vi "Start and End to Array.vi"(4 "Round Factor":dbl=1000000000.0, 5 "Step":dbl=0.1, 6 "End":dbl=2.0, 7 "Start":dbl=-0.5) -> (1 "Array":dbl[](array[numeric])=[-0.5, -0.4, -0.3, -0.2, -0.1, 0.0, 0.1, 0.2, 0.3, 0.4, 0.5, 0.6, 0.7, 0.8, 0.9, 1.0, 1.1, 1.2, 1.3, 1.4, 1.5, 1.6, 1.7, 1.8, 1.9, 2.0])   [LabVIEW 2010]
panel:
  in  "Sweep Style":enum16{"Linear", "Log"}(ring)
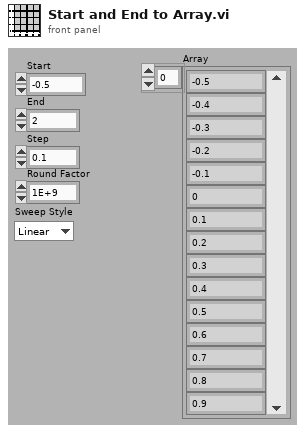
[diagram p1: front panel]
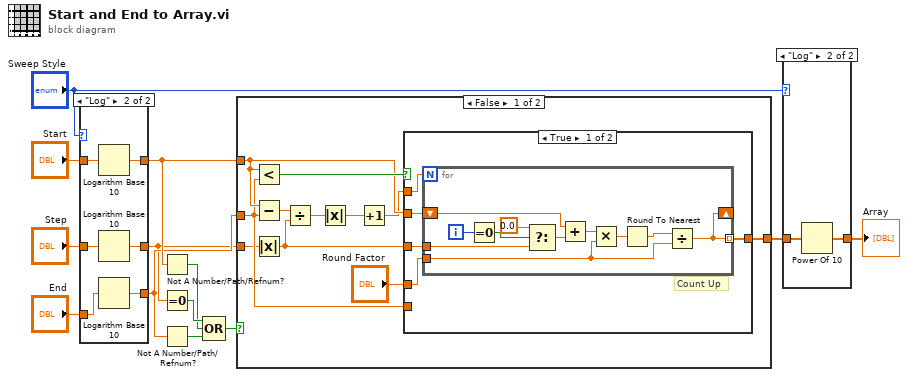
[diagram p0: block diagram]
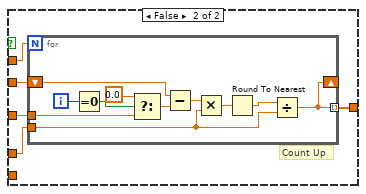
[diagram p4: hidden frame]
diagram:
  n1 = case shown="\"Log\"" "Sweep Style" {
    tunnel: "Start" -> [w16 w22]
    tunnel: [w16 w21] -> w8
    tunnel: "End" -> [w15 w18]
    tunnel: [w15 w17] -> w6
    tunnel: "Step" -> [w14 w20]
    tunnel: [w14 w19] -> w4
    frame "Linear", Default {
    }
    frame "Log" {
      n2 = Logarithm Base 10(1:w22) -> (0:w21:dbl)
      n3 = Logarithm Base 10(1:w20) -> (0:w19:dbl)
      n4 = Logarithm Base 10(1:w18) -> (0:w17:dbl)
    }
  }
  n5 = Not A Number/Path/Refnum?(number/path/refnum=w8) -> (NaN/Path/Refnum?=w12:bool)
  n6 = Equal To 0?(x=w4) -> (x = 0?=w13:bool)
  n7 = Not A Number/Path/Refnum?(number/path/refnum=w6) -> (NaN/Path/Refnum?=w11:bool)
  n8 = Compound Arithmetic op=OR(w13, w12, w11) -> (w10:bool)
  n9 = case shown="False" w10 {
    tunnel: w8 -> [w32 _]
    tunnel: w6 -> [w31 _]
    tunnel: w4 -> [w25 _]
    tunnel: [w23 _] -> w3
    frame False {
      n10 = Less?(x=w32, y=w31) -> (x < y?=w33:bool)
      n11 = Subtract(x=w32, y=w31) -> (x-y=w30:dbl)
      n12 = Absolute Value(x=w25) -> (abs(x)=w24:dbl)
      n13 = Divide(x=w30, y=w24) -> (x/y=w29:dbl)
      n14 = Absolute Value(x=w29) -> (abs(x)=w28:dbl)
      n15 = Increment(x=w28) -> (x+1=w27:dbl)
      n16 = case shown="True" w33 {
        tunnel: w32 -> [w35 w51]
        tunnel: w24 -> [w38 w54]
        tunnel: [w37 w53] -> w23
        tunnel: w31 -> [_ _]
        tunnel: w27 -> [w36 w52]
        tunnel: "Round Factor" -> [w34 w50]
        frame True {
          # "Count Up"
          n17 = for {
            N: w36 -> [_]
            tunnel: w38 -> [w45]
            tunnel: [w40] -> w37 mode=indexing
            shift-right: [w40] -> _
            shift-left: w35 -> [w49]
            tunnel: w34 -> [w39]
            i -> [w48]
            n18 = Equal To 0?(x=w48) -> (x = 0?=w47:bool)
            n19 = Select(t=0.0, s=w47, f=w45) -> (s? t:f=w44:dbl)
            n20 = Add(x=w49, y=w44) -> (x+y=w41:dbl)
            n21 = Multiply(x=w41, y=w39) -> (x*y=w43:dbl)
            n22 = Round To Nearest(number=w43) -> (nearest integer value=w42:dbl)
            n23 = Divide(x=w42, y=w39) -> (x/y=w40:dbl)
          }
        }
        frame False {
          # "Count Up"
          n24 = for {
            N: w52 -> [_]
            tunnel: w54 -> [w61]
            tunnel: [w56] -> w53 mode=indexing
            shift-right: [w56] -> _
            shift-left: w51 -> [w65]
            tunnel: w50 -> [w55]
            i -> [w64]
            n25 = Equal To 0?(x=w64) -> (x = 0?=w63:bool)
            n26 = Select(t=0.0, s=w63, f=w61) -> (s? t:f=w60:dbl)
            n27 = Subtract(x=w65, y=w60) -> (x-y=w57:dbl)
            n28 = Multiply(x=w57, y=w55) -> (x*y=w59:dbl)
            n29 = Round To Nearest(number=w59) -> (nearest integer value=w58:dbl)
            n30 = Divide(x=w58, y=w55) -> (x/y=w56:dbl)
          }
        }
      }
    }
    frame True {
    }
  }
  n31 = case shown="\"Log\"" "Sweep Style" {
    tunnel: w3 -> [w66 w68]
    tunnel: [w66 w67] -> w1
    frame "Linear", Default {
    }
    frame "Log" {
      n32 = Power Of 10(x=w68) -> (10^x=w67:dbl[])
    }
  }
  "Array" <- w1
